vi "NotificationBar.vi"(9 "NotificationBarString":string) -> ()   [LabVIEW 2012]
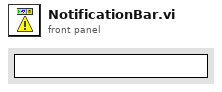
[diagram p1: front panel]
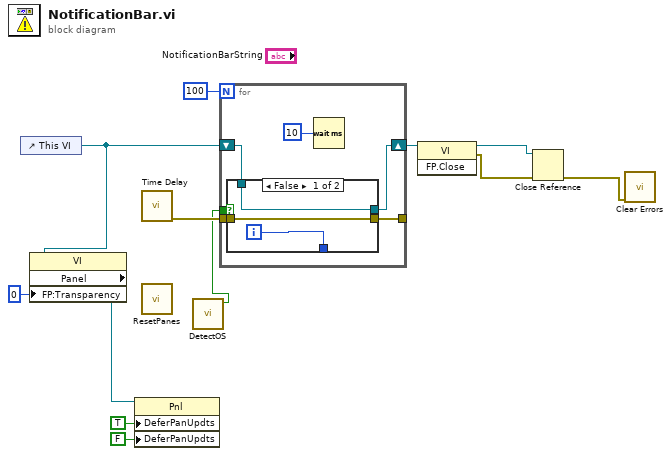
[diagram p0: block diagram]
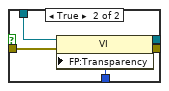
[diagram p2: hidden frame]
diagram:
  n1 = control-ref of="This VI"() -> (w6:refnum<vi>)
  n2 = property class="VI"(reference=w6, "FP:Transparency"=u8 0 ("Front Panel Window:Transparency")) -> ("Panel"=w5:refnum<vi>)  [unwired: 1 in, 2 out]
  n3 = property class="Pnl"(reference=w5, "DeferPanUpdts"=TRUE ("Defer Panel Updates"), "DeferPanUpdts"=FALSE ("Defer Panel Updates")) -> ()  [unwired: 1 in, 2 out]
  n4 = call "Time Delay"() -> ("error out"=w10:errorcluster)  [unwired: 11 in]
  n5 = call "ResetPanes.vi"() -> ()  [unwired: 12 in]
  n6 = call "DetectOS.vi"() -> ("XP?"=w1:bool)  [unwired: 11 in]
  n7 = for {
    N: 100 -> [_]
    tunnel: w10 -> [w16]
    shift-right: [w15] -> w11
    shift-left: w6 -> [w19]
    tunnel: [w14] -> _
    tunnel: w1 -> [w13]
    i -> [w18]
    n8 = case shown="False" w13 {
      tunnel: w19 -> [w21 w26]
      tunnel: w18 -> [_ w25]
      tunnel: w16 -> [w20 w24]
      tunnel: [w21 w23] -> w15
      tunnel: [w20 w22] -> w14
      frame False {
      }
      frame True {
        n9 = property class="VI"(reference=w26, error in=w24, "FP:Transparency"=w25) -> (reference out=w23:refnum<vi>, error out=w22:errorcluster)
      }
    }
    n10 = Wait (ms)(milliseconds to wait=u32 10) -> ()  [unwired: 1 out]
  }
  n11 = invoke class="VI" method="FP.Close"(reference=w11) -> (reference out=w9:refnum<vi>, error out=w8:errorcluster)  [unwired: 2 in, 1 out]
  n12 = Close Reference(reference=w9, error in (no error)=w8) -> (error out=w7:errorcluster)
  n13 = call <vilib>:"Clear Errors.vi"("error in (no error)"=w7) -> ()  [unwired: 5 in, 2 out]
